vi "Test Formatting Panel Template.vi"(4 "error in (no error)":errorcluster, 6 "Format Cache TDM":path, 7 "Template container ref (NULL)":refnum<k20>) -> (0 "error out":errorcluster)   [LabVIEW 2011]
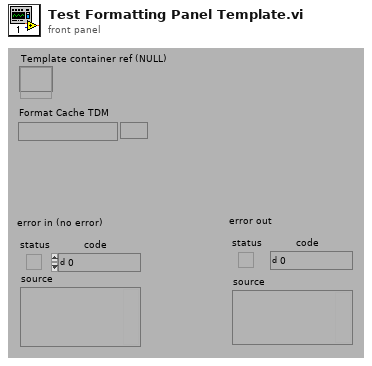
[diagram p1: front panel]
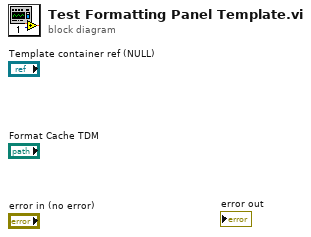
[diagram p0: block diagram]
diagram:
